vi "Update_Position_Perform_ColDet.vi"(5 "Background Alpha":dbl=0.5, 7 "Background Color":u32(colorbox)=13750737, 8 "error in":errorcluster, 9 "Number Static":i32, 10 "Moving Position Array":T1[](array[typedef]), 11 "Probe Position":T1) -> (0 "error out":errorcluster, 2 "Collision Detected Array":bool[](array[boolean]), 3 "Separation Distance Array":T2[](array[typedef]))   [LabVIEW 2011]
doc: "This VI performs the collision detection between the probe and the moving and static geometry. Note that collision is never detected between the moving and static geometry, only the probe and static geometry. Returns an array of separation distances and collision booleans, between the probe and each object (moving then static."
uses:
  SObject.ctl
  Vector3D.ctl
  Enflo_Collision_Detection.dll
  <vilib>/picture/3D Picture Control/NI_3D Picture Control.lvlib
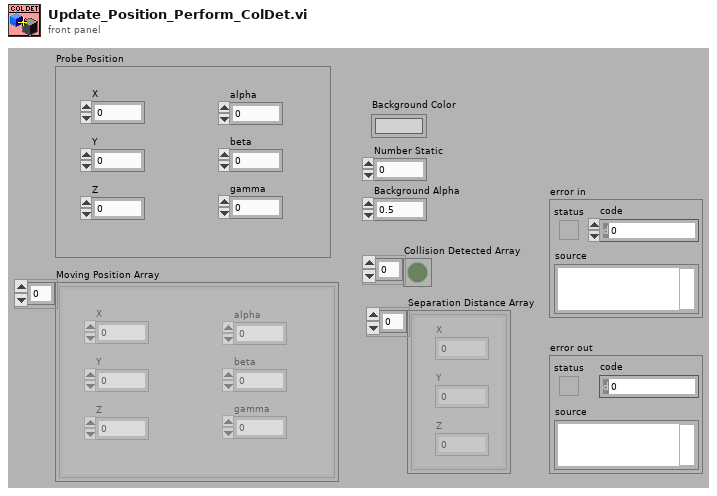
[diagram p1: front panel]
types:
  T1 = typedef "SObject.ctl" = cluster{"X":dbl, "Y":dbl, "Z":dbl, "alpha":dbl, "beta":dbl, "gamma":dbl}
  T2 = typedef "Vector3D.ctl" = cluster{"X":dbl, "Y":dbl, "Z":dbl}
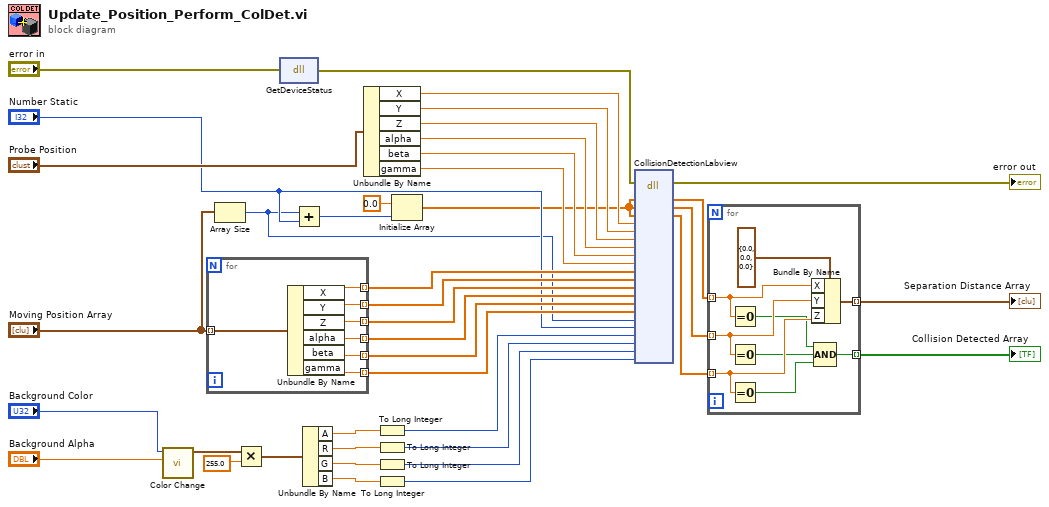
[diagram p0: block diagram]
diagram:
  n1 = call <vilib>:"Color Change.vi"("Alpha"="Background Alpha", "Color"="Background Color") -> ("RGBA"=w17:cluster{"R":sgl, "G":sgl, "B":sgl, "A":sgl})  [unwired: 9 in]
  n2 = for {
    tunnel: "Moving Position Array" -> [w47] mode=indexing
    tunnel: [w46] -> w35 mode=indexing
    tunnel: [w45] -> w36 mode=indexing
    tunnel: [w44] -> w37 mode=indexing
    tunnel: [w43] -> w38 mode=indexing
    tunnel: [w42] -> w39 mode=indexing
    tunnel: [w41] -> w40 mode=indexing
    n3 = Unbundle By Name(w47) -> ("X"=w46:dbl, "Y"=w45:dbl, "Z"=w44:dbl, "alpha"=w43:dbl, "beta"=w42:dbl, "gamma"=w41:dbl)
  }
  n4 = Array Size(array="Moving Position Array") -> (size(s)=w5:i32)
  n5 = Multiply(x=w17, y=sgl 255.0 ("R")) -> (x*y=w15:cluster{"R":sgl, "G":sgl, "B":sgl, "A":sgl})
  n6 = dll-call lib="C:/Users/Nick/Desktop/Release/Enflo_Collision_Detection.dll" fn="GetDeviceStatus"(error in="error in") -> (error out=w1:errorcluster)  [unwired: 3 in, 1 out]
  n7 = Add(x=w5, y="Number Static") -> (x+y=w4:i32)
  n8 = Unbundle By Name(w15) -> ("A"=w8:sgl, "R"=w12:sgl, "G"=w13:sgl, "B"=w14:sgl)
  n9 = Unbundle By Name("Probe Position") -> ("X"=w29:dbl, "Y"=w30:dbl, "Z"=w31:dbl, "alpha"=w32:dbl, "beta"=w33:dbl, "gamma"=w34:dbl)
  n10 = To Long Integer(number=w8) -> (32bit integer=w7:i32)
  n11 = To Long Integer(number=w12) -> (32bit integer=w11:i32)
  n12 = To Long Integer(number=w13) -> (32bit integer=w10:i32)
  n13 = To Long Integer(number=w14) -> (32bit integer=w9:i32)
  n14 = Initialize Array(0.0 ("element"), w4) -> (w20:dbl[])
  n15 = dll-call lib="C:/Users/Nick/Desktop/Release/Enflo_Collision_Detection.dll" fn="CollisionDetectionLabview"(error in=w1, "SepDistX"=w20, "SepDistY"=w20, "SepDistZ"=w20, "ProbePosX"=w29, "ProbePosY"=w30, "ProbePosZ"=w31, "ProbeRotX"=w32, "ProbeRotY"=w33, "ProbeRotZ"=w34, "Moving Pos X"=w35, "Moving Pos Y"=w36, "Moving Pos Z"=w37, "Moving Rot X"=w38, "Moving Rot Y"=w39, "Moving Rot Z"=w40, "NumMoving"=w5, "NumStatic"="Number Static", "A"=w7, "R"=w11, "G"=w10, "B"=w9) -> (error out=→"error out":errorcluster, "SepDistX"=w24:dbl[], "SepDistY"=w25:dbl[], "SepDistZ"=w26:dbl[])  [unwired: 21 in, 1 out]
  n16 = for {
    tunnel: w24 -> [w54] mode=indexing
    tunnel: w25 -> [w53] mode=indexing
    tunnel: w26 -> [w52] mode=indexing
    tunnel: [w56] -> w27 mode=indexing
    tunnel: [w48] -> w3 mode=indexing
    n17 = Equal To 0?(x=w54) -> (x = 0?=w51:bool)
    n18 = Equal To 0?(x=w53) -> (x = 0?=w50:bool)
    n19 = Equal To 0?(x=w52) -> (x = 0?=w49:bool)
    n20 = Bundle By Name(cluster=T2 {"X"=0.0, "Y"=0.0, "Z"=0.0} ("SepDist"), "X"=w54, "Y"=w53, "Z"=w52) -> (w56:T2)
    n21 = Compound Arithmetic op=AND(w51, w50, w49) -> (w48:bool)
  }
  "Separation Distance Array" <- w27
  "Collision Detected Array" <- w3
